vi "振动试验server.vi"() -> ()   [LabVIEW 2010]
uses:
  频率.vi
  Instance          10 22Saved   振动试验server .vi
  Instance           1 22Saved   振动试验server .vi
  <vilib>/Analysis/3filter.llb/Butterworth Filter (DBL).vi
  <vilib>/Analysis/4window.llb/Hanning Window (DBL).vi
  <vilib>/Utility/file.llb/Write To Spreadsheet File (DBL).vi
  <vilib>/Analysis/NI_AALPro.lvlib
  <vilib>/Analysis/NI_AALBase.lvlib
panel:
  in  "查看结果":bool
  in  "记录数据":bool
  in  "实验编号":string="001"
  in  "传感器电压灵敏度":dbl=0.151 format="%.3f"
  out "网络传输错误":bool
  in  "采样数(s)":i32=1024
  out "加速度信号(m/ss)":dbl[](graph)
  in  "关闭":bool
  out "频  率(Hz)":T1(graph)={0, "df"=inf, "Power Spectrum (V^2 rms)"=[]}
  out "频  率":dbl=nan format="%.4f"
  in  "采样率(S/s)":dbl=2048.0
  # "振 动 实 验 服 务 器"
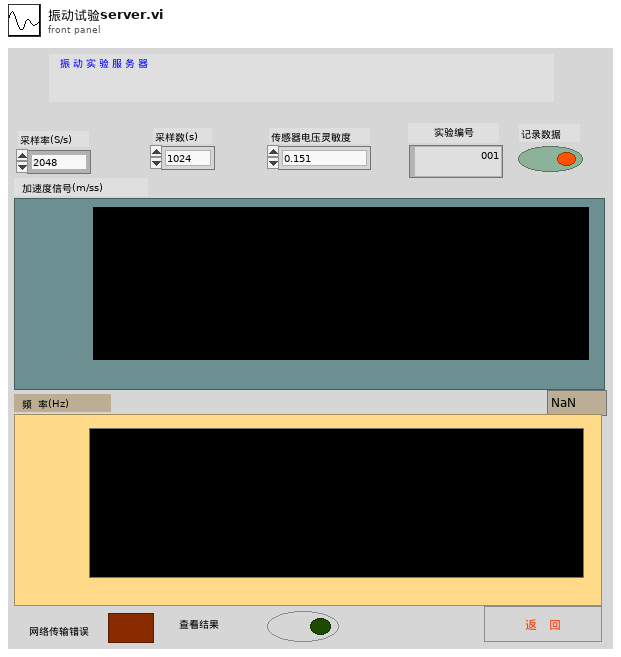
[diagram p1: front panel]
types:
  T1 = cluster{i32, "df":dbl, "Power Spectrum (V^2 rms)":dbl[]}
  T2 = enum32{"Lowpass", "Highpass", "Bandpass", "Bandstop"}
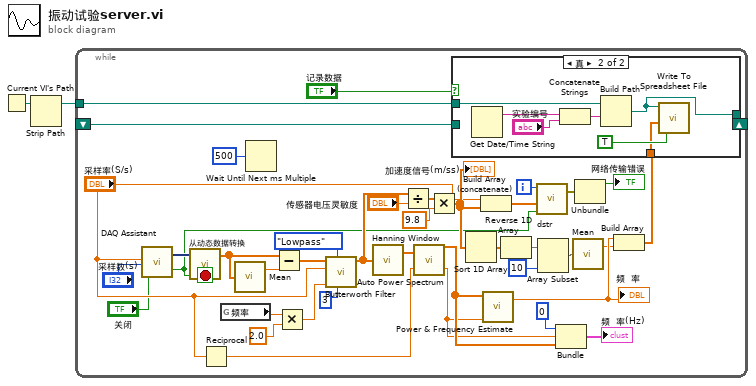
[diagram p0: block diagram]
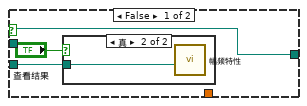
[diagram p2: hidden frame]
diagram:
  n1 = Current VI's Path() -> (path=w2:path)
  n2 = Strip Path(path=w2) -> (stripped path=w1:path)  [unwired: 1 out]
  n3 = while {
    tunnel: w1 -> [w26]
    shift-right: [w22] -> _
    shift-left: _ -> [w21]
    i -> [w15]
    stop <- w3 stop-if-true
    n4 = call "DAQ Assistant"("rate"="采样率(S/s)", "number of samples"="采样数(s)", "stop (F)"="关闭") -> ("data"=w7:dynamicdata, "stopped"=w3:bool)  [unwired: 13 in, 2 out]
    n5 = call "从动态数据转换"("Dynamic Data Type"=w7) -> ("Array"=w6:dbl[])  [unwired: 3 in]
    n6 = Reciprocal(x="采样率(S/s)") -> (1/x=w42:dbl)
    n7 = global read "频率.vi" "频率"() -> (w8:dbl)
    n8 = call <vilib>:"Mean.vi"("X"=w6) -> ("mean"=w33:dbl)  [unwired: 1 out]
    n9 = Wait Until Next ms Multiple(millisecond multiple=u32 500 ("毫秒倍数")) -> ()  [unwired: 1 out]
    n10 = Subtract(x=w6, y=w33) -> (x-y=w32:dbl[])
    n11 = Multiply(x=w8, y=2.0) -> (x*y=w29:dbl)
    n12 = call-poly <vilib>:"Butterworth Filter.vi"("order"=3, "filter type"=T2."Lowpass", "low cutoff freq: fl"=w29, "sampling freq: fs"="采样率(S/s)", "X"=w32) -> ("Filtered X"=w31:dbl[])  [unwired: 3 in, 1 out]
    n13 = call-poly <vilib>:"Hanning Window.vi"("X"=w31) -> ("Windowed X"=w41:dbl[])  [unwired: 1 out]
    n14 = Divide(x=w31, y="传感器电压灵敏度") -> (x/y=w35:dbl[])
    n15 = call <vilib>:"Auto Power Spectrum.vi"("dt"=w42, "Signal (V)"=w41) -> ("df"=w39:dbl, "Power Spectrum (V^2 rms)"=w40:dbl[])
    n16 = Multiply(x=w35, y=9.8) -> (x*y=w12:dbl[])
    "加速度信号(m/ss)" <- w12
    n17 = Sort 1D Array(array=w12) -> (sorted array=w14:dbl[])
    n18 = Build Array (concatenate)("采样率(S/s)", w12) -> (w20:dbl[])
    n19 = call <vilib>:"Power & Frequency Estimate.vi"("df"=w39, "Power Spectrum (V^2 rms)"=w40) -> ("est frequency peak"=w24:dbl)  [unwired: 4 in, 1 out]
    "频  率" <- w24
    n20 = Reverse 1D Array(array=w14) -> (reversed array=w13:dbl[])
    n21 = call "dstr.vi"("stop"=w3, "data"=w20, "i"=w15) -> ("error out"=w19:errorcluster)  [unwired: 1 in, 1 out]
    n22 = Array Subset(array=w13, length=10) -> (w17:dbl[])  [unwired: 1 in]
    n23 = Bundle(0, "df"=w39, "Power Spectrum (V^2 rms)"=w40) -> (→"频  率(Hz)":T1)  [unwired: 1 in]
    n24 = call <vilib>:"Mean.vi"("X"=w17) -> ("mean"=w16:dbl)  [unwired: 1 out]
    n25 = Unbundle(w19) -> ("status"=→"网络传输错误":bool)  [unwired: 2 out]
    n26 = Build Array(w24, w16) -> (w23:dbl[])
    n27 = case shown="真" "记录数据" {
      tunnel: w26 -> [_ w47]
      tunnel: w23 -> [_ w51]
      tunnel: [w43 w46] -> w22
      tunnel: w21 -> [w43 _]
      frame False {
        n28 = case shown="真" "查看结果" {
          tunnel: w43 -> [_ w45]
          frame False {
          }
          frame True {
            n29 = call "幅频特性.vi"("file path (dialog if empty)"=w45) -> ()  [unwired: 1 in]
          }
        }
      }
      frame True {
        n30 = Get Date/Time String() -> (date string=w49:string)  [unwired: 3 in, 1 out]
        n31 = Concatenate Strings(w49, "实验编号") -> (w48:string)
        n32 = Build Path(base path=w47, name or relative path=w48) -> (appended path=w46:path)
        n33 = call-poly <vilib>:"Write To Spreadsheet File.vi"("append to file? (new file:F)"=TRUE, "1D data"=w51, "file path (dialog if empty)"=w46) -> ()  [unwired: 5 in, 1 out]
      }
    }
  }
